vi "DDL_Query.vi"(0 "System no.":i32=1 min=1 max=4 step=1, 2 "Table no.":i32=1, 3 "Offset":i32=1, 4 "N":i32=100, 5 "error in":errorcluster) -> (14 "Values":dbl[](array[numeric]) format="%.6f", 15 "DDL? string":string, 19 "error out":errorcluster)   [LabVIEW 2020]
doc: "Returns N values from specified DDL Table (in the controller memory). For large N values, communication timeout must be set long enough, otherwise a comm. error may occur.\n\nE-710: Table number can be 1 to 8. First stored value in table has index 1, index 0 is the DDL repeat number. Maximum 32768 values can be stored.\n\nE-712: Table number can be 1 to the maximum number of axes (query with TLT? for the number of DDL tables). Offset is start point and must be greater than zero, because first stored value in table has index 1. Maximum 262,144 values can be stored.\n\nE-725, E-727: Table number can be 1 to the maximum number of axes (query with TLT? for the number of DDL tables). Offset is start point and must be greater than zero, because first stored value in table has index 1. Maximum 262,144 values can be stored.\n\nE-753: Table number can be 1. Offset is start point and must be greater than zero, because first stored value in table has index 1. Maximum 65,536 values can be stored.\n\nE-754: Table number can be 1. Offset is start point and must be greater than zero, because first stored value in table has index 1. Maximum 1,046,076 values can be stored."
uses:
  Syntax.ctl
  Global1.vi
panel:
  # "Returns N values from specified DDL Table (in the controller memory). For large N values, communication timeout must be set long enough, otherwise a comm.error may occur."
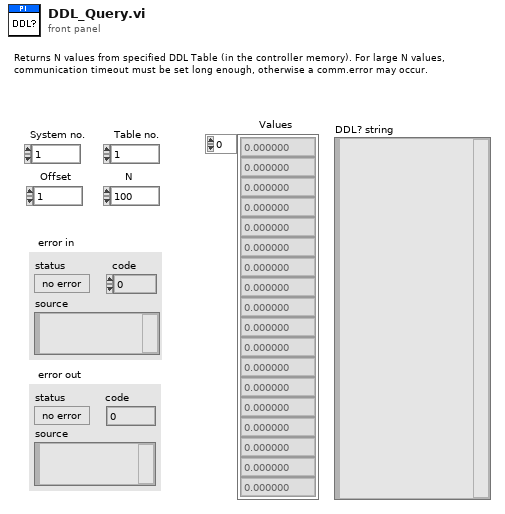
[diagram p1: front panel]
types:
  T1 = typedef "Syntax.ctl" = enum16{"GCS 1.0", "GCS 2.0", "GCS 3.0"}
  T2 = cluster{"Read (F)/Write":bool, "Path":path, "Datastream":string, "ArrayName":string}
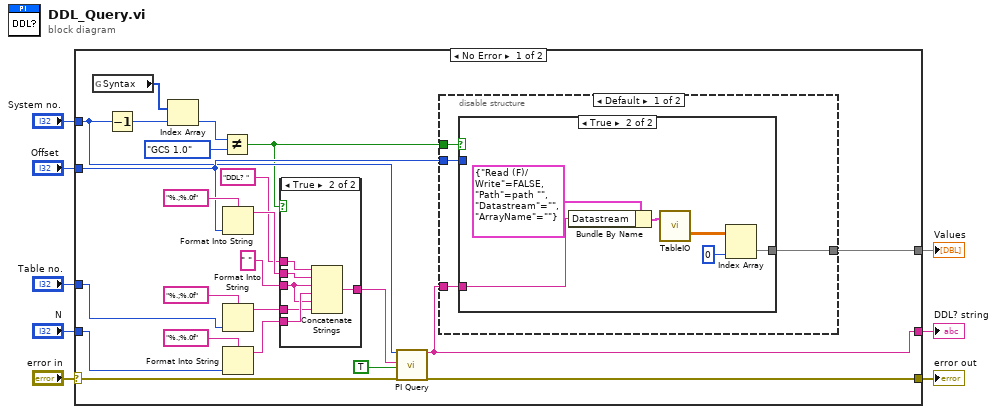
[diagram p0: block diagram]
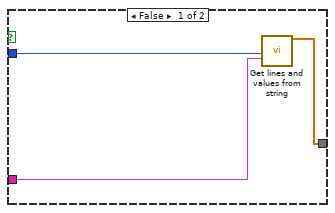
[diagram p2: hidden frame]
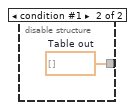
[diagram p3: hidden frame]
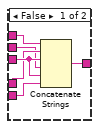
[diagram p4: hidden frame]
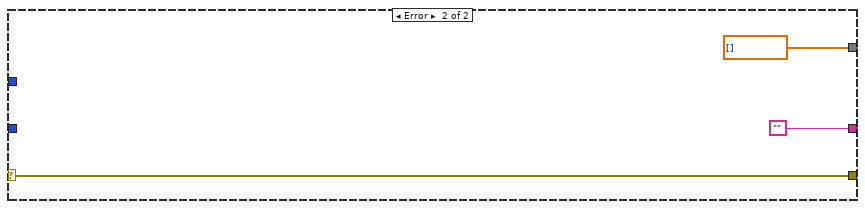
[diagram p5: hidden frame]
diagram:
  n1 = case shown="No Error" "error in" {
    selector: "error in" -> [w10 w58]
    tunnel: "System no." -> [w14 _]
    tunnel: [w12 w58] -> w7
    tunnel: [w30 dbl[] []] -> w6
    tunnel: "Offset" -> [w29 _]
    tunnel: "Table no." -> [w27 _]
    tunnel: "N" -> [w21 _]
    tunnel: [w11 ""] -> w2
    frame No Error {
      n2 = global read "Global1.vi" "Syntax"() -> (w15:T1[])
      n3 = Decrement(x=w14) -> (x-1=w16:i32)
      n4 = Index Array(array=w15, index=w16) -> (element=w17:T1)
      n5 = Not Equal?(x=w17, y=Syntax."GCS 1.0") -> (x != y?=w13:bool)
      n6 = Format Into String(format string="%.;%.0f" ("Format String"), w29) -> (resulting string=w23:string)  [unwired: 2 in, 1 out]
      n7 = Format Into String(format string="%.;%.0f" ("Format String"), w27) -> (resulting string=w25:string)  [unwired: 2 in, 1 out]
      n8 = Format Into String(format string="%.;%.0f" ("Format String"), w21) -> (resulting string=w22:string)  [unwired: 2 in, 1 out]
      n9 = case shown="True" w13 {
        tunnel: " " -> [w51 w53]
        tunnel: w25 -> [w50 w52]
        tunnel: w23 -> [w49 w55]
        tunnel: w22 -> [w48 w54]
        tunnel: "DDL? " -> [w47 w57]
        tunnel: [w46 w56] -> w19
        frame False {
          n10 = Concatenate Strings(w47, w50, w51, w49, w51, w48) -> (w46:string)
        }
        frame True {
          n11 = Concatenate Strings(w57, w55, w53, w54, w53, w52) -> (w56:string)
        }
      }
      n12 = call "PI Query.vi"("System no."=w14, "String to send"=w19, "Attach termination char.?"=TRUE ("Attach Linefeed?"), "error in"=w10) -> ("String read"=w11:string, "error out"=w12:errorcluster)  [unwired: 3 in, 11 out]
      n13 = disable-structure shown="Default" {
        disable-tunnel: [w35 w45] -> w30
        disable-tunnel: w29 -> [w34 _]
        disable-tunnel: w13 -> [w33 _]
        disable-tunnel: w11 -> [w32 _]
        frame condition #0 (active) {
          n14 = case shown="True" w33 {
            tunnel: [w38 w41] -> w35
            tunnel: w34 -> [w37 _]
            tunnel: w32 -> [w36 w40]
            frame False {
              n15 = call "Get lines and values from string.vi"("Array size"=w37, "Input string"=w36) -> ("Numerical values"=w38:dbl[])  [unwired: 17 out]
            }
            frame True {
              n16 = Bundle By Name(cluster=T2 {"Read (F)/Write"=FALSE, "Path"=path "", "Datastream"="", "ArrayName"=""} ("IOSource"), "Datastream"=w40) -> (w44:T2)
              n17 = call "TableIO.vi"("IOSource"=w44) -> ("Table out"=w42:dbl[][])  [unwired: 5 in, 13 out]
              n18 = Index Array(array=w42, index (col)=0 ("index (row)")) -> (element=w41:dbl[])  [unwired: 1 in]
            }
          }
        }
        frame condition #1 {
          w45 = dbl[] []  # Table out
        }
      }
    }
    frame Error {
    }
  }
  "error out" <- w7
  "Values" <- w6
  "DDL? string" <- w2
